vi "Navigation Loop.vi"(8 "error in (no error)":errorcluster) -> (0 "error out":errorcluster)   [LabVIEW 2016]
uses:
  Typedef/Filter Data.ctl
  <vilib>/Platform/TimedLoop/XDataNode/timing_clust.ctl
  <vilib>/Platform/TimedLoop/XDataNode/nitl_modes.ctl
  <vilib>/Platform/TimedLoop/XDataNode/wakeup.ctl
  <vilib>/Analysis/coordinate.llb/Wrap Angle (scalar).vi
  <vilib>/Analysis/baseanly.llb/Real Dot Product.vi
  <vilib>/Utility/file.llb/Read Delimited Spreadsheet (DBL).vi
  <vilib>/Utility/error.llb/Error Cluster From Error Code.vi
  Shared resoruces/Front Panel Control Variables.vi
  Shared resoruces/Navigation Variables.vi
  <vilib>/addons/control/pid/pid.llb/PID (DBL).vi
  <vilib>/ErrorRing/Error Ring.xnode
  <vilib>/platform/TimedLoop/XDataNode/XDataNode.xnode
  <vilib>/Platform/TimedLoop/XDataNode/XDNodeRunTimeDep.lvlib
  Shared resoruces/Shared resources RT.lvlib
  <vilib>/addons/control/pid/NI_PID_pid.lvlib
  <vilib>/Analysis/NI_AALBase.lvlib
  <vilib>/Analysis/NI_AAL_Angle.lvlib
  <vilib>/ptbypt/NI_PtbyPt.lvlib
panel:
  in  "Reference position":cluster{"Lat":dbl, "Long":dbl}={"Lat"=57.731096, "Long"=12.086851}
  in  "Heading PID gains":T1={"proportional gain (Kc)"=0.2, "integral time (Ti, min)"=0.0, "derivative time (Td, min)"=0.0} {"derivative time (Td, min)" format="%.3f"; "integral time (Ti, min)" format="%.3f"; "proportional gain (Kc)" format="%.3f"}
  in  "Lateral PID Gains":T1={"proportional gain (Kc)"=5.0, "integral time (Ti, min)"=600.0, "derivative time (Td, min)"=0.0} {"derivative time (Td, min)" format="%.3f"; "integral time (Ti, min)" format="%.3f"; "proportional gain (Kc)" format="%.3f"}
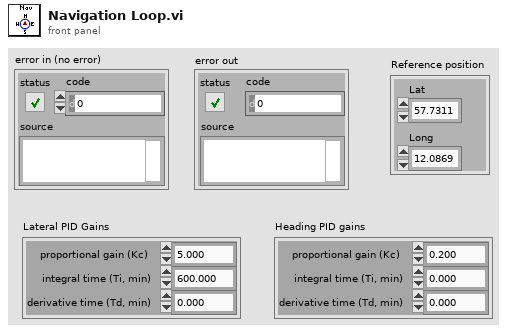
[diagram p1: front panel]
types:
  T1 = cluster{"proportional gain (Kc)":dbl, "integral time (Ti, min)":dbl, "derivative time (Td, min)":dbl}
  T2 = typedef "Filter Data.ctl" = cluster{"Yaw":dbl, "Lat":dbl, "Long":dbl}
  T3 = typedef "XDNodeRunTimeDep.lvlib/timing_clust.ctl" = cluster{"Expected End [f-1]":u64, "Actual End [f-1]":u64, "Finished Late? [f-1]":bool, "Expected End [i-1]":u64, "Actual End [i-1]":u64, "Finished Late? [i-1]":bool, "Expected Start [i]":u64, "Actual Start [i]":u64, "Expected Start [f]":u64, "Actual Start [f]":u64, "Source Name":string, "Structure Name":string, "Period":i64, "Deadline":i64, "Offset":i64, "Start":i64, "Priority":i32, "Timeout":i32, "Mode":T4, "Wakeup Reason":T5, "Error":errorcluster, "Source Type":string, "Secondary Source Type":string, "Global End Time":u64, "Global Start Time":u64, "Frame Duration":u64, "Iteration Duration":u64, "Assigned CPU":i32, "I/O Scan Engine Mode":u32}
  T4 = typedef "XDNodeRunTimeDep.lvlib/nitl_modes.ctl" = enum32{"No Change", "Process missed periods, maintain original phase", "Discard missed periods, maintain original phase", "Process missed periods, ignore original phase", "Discard missed periods, ignore original phase"}
  T5 = typedef "XDNodeRunTimeDep.lvlib/wakeup.ctl" = enum32{"Normal", "Aborted", "Asynchronous wakeup", "Timing source error", "Timed loop error", "Timeout"}
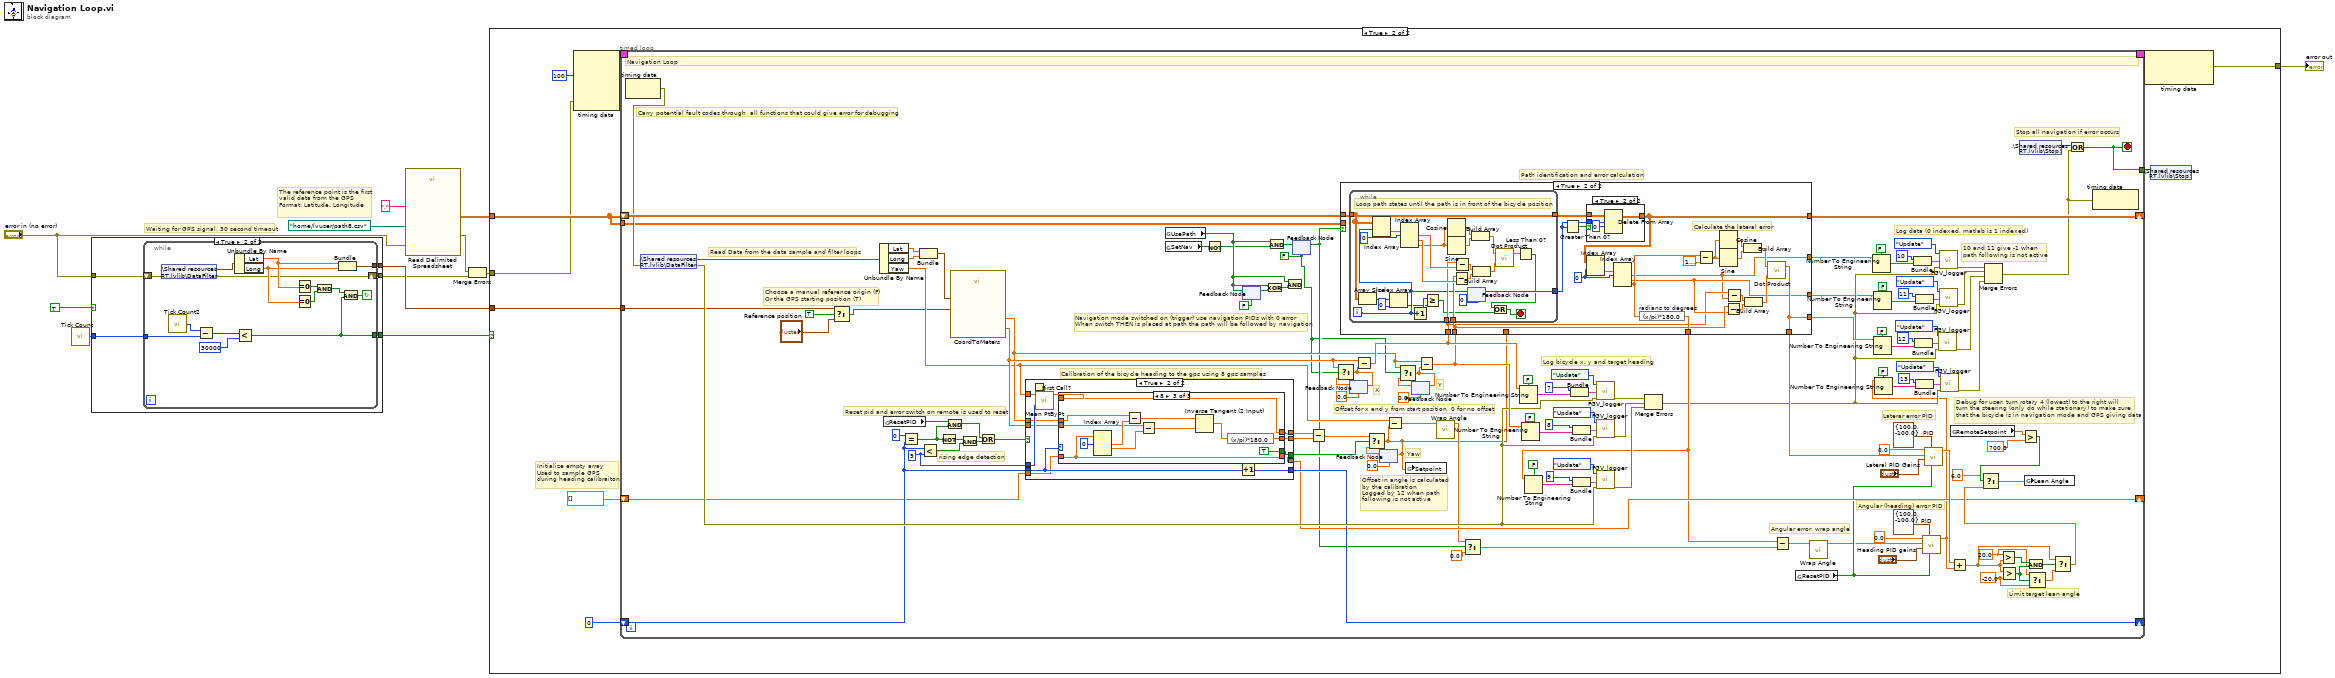
[diagram p0: block diagram]
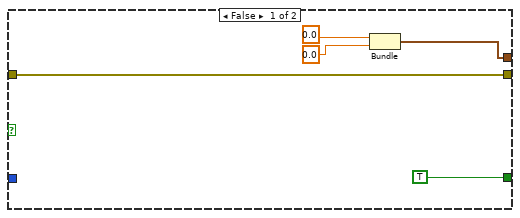
[diagram p2: hidden frame]
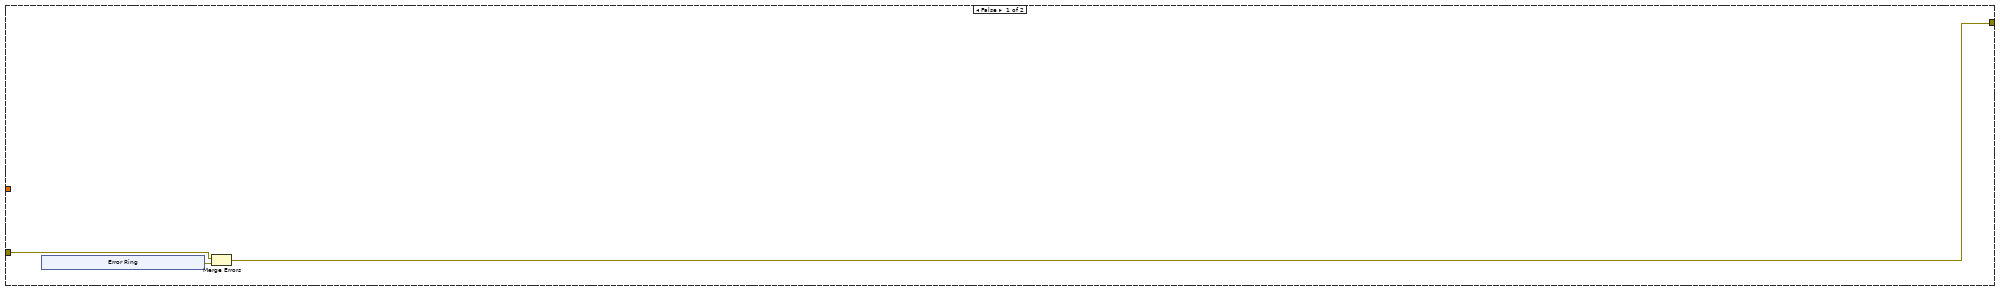
[diagram p3: hidden frame]
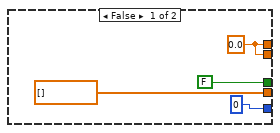
[diagram p4: hidden frame]
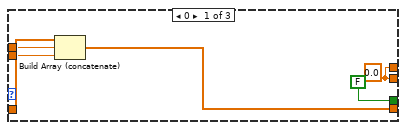
[diagram p5: hidden frame]
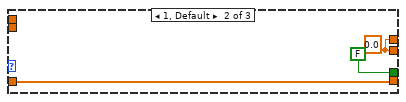
[diagram p6: hidden frame]
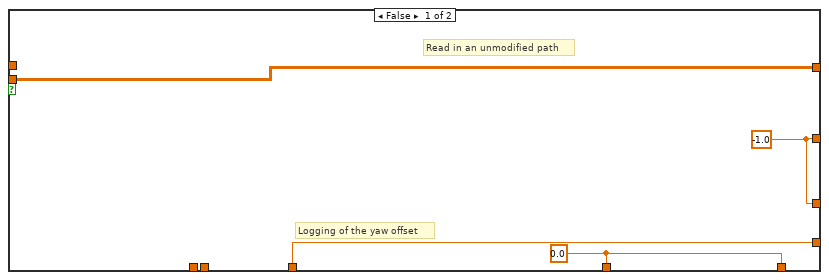
[diagram p7: hidden frame]
diagram:
  # "Waiting for GPS signal, 30 second timeout"
  # "The reference point is the first valid data from the GPS\nFormat: Latitude, Longitude"
  n1 = call "Tick Count"() -> ("Tick Count(mSec)"=w3:u32)
  n2 = case shown="True" TRUE {
    tunnel: "error in (no error)" -> [w17 w22]
    tunnel: [w16 w21] -> w10
    tunnel: [w17 w20] -> w7
    tunnel: w3 -> [_ w19]
    tunnel: [TRUE w18] -> w1
    frame False {
      n3 = Bundle(0.0, 0.0) -> (w16:cluster{dbl, dbl})  [unwired: 1 in]
    }
    frame True {
      n4 = while {
        shift-right: [w31] -> w20
        shift-left: w22 -> [w30]
        tunnel: [w34] -> w21
        tunnel: w19 -> [w26]
        tunnel: [w23] -> w18
        stop <- w28 continue-if-true
        n5 = shared-variable ".\\Shared resources RT.lvlib\\DataFilter"(error in=w30) -> (w35:T2, error out=w31:errorcluster)
        n6 = call "Tick Count2"() -> ("Tick Count(mSec)"=w27:u32)
        n7 = Subtract(x=w27, y=w26) -> (x-y=w25:u32)
        n8 = Unbundle By Name(w35) -> ("Lat"=w33:dbl, "Long"=w32:dbl)
        n9 = Less?(x=w25, y=u32 30000) -> (x < y?=w23:bool)
        n10 = Equal To 0?(x=w33) -> (x = 0?=w37:bool)
        n11 = Equal To 0?(x=w32) -> (x = 0?=w36:bool)
        n12 = And(x=w37, y=w36) -> (x .and. y?=w29:bool)
        n13 = Bundle("Lat"=w33, "Long"=w32) -> (w34:cluster{"Lat":dbl, "Long":dbl})  [unwired: 1 in]
        n14 = And(x=w29, y=w23) -> (x .and. y?=w28:bool)
      }
    }
  }
  n15 = call-poly <vilib>:"Read Delimited Spreadsheet.vi"("file path (dialog if empty)"=path "/home/lvuser/path8.csv", "error in (no error)"="error in (no error)", "delimiter (\\t)"="," ("delimiter (\\t)")) -> ("all rows"=w6:dbl[][], "error out"=w8:errorcluster)  [unwired: 7 in, 4 out]
  n16 = Merge Errors(w8, w7) -> (w9:errorcluster)
  n17 = case shown="True" w1 {
    tunnel: [w38 w49] -> w11
    tunnel: w10 -> [_ w53]
    tunnel: w9 -> [w40 w50]
    tunnel: w6 -> [_ w51]
    frame False {
      n18 = xnode "Error Ring"() -> ("error out"=w39:errorcluster)
      n19 = Merge Errors(w40, w39) -> (w38:errorcluster)
    }
    frame True {
      # "Initialize empty array\nUsed to sample GPS \nduring heading calibraiton"
      n20 = node-c288(i64 100 ("Period"), w50) -> (w55:T3)  [unwired: 3 in]
      n21 = timed-loop {
        shift-right: [w187] -> _
        shift-left: w51 -> [w186]
        tunnel: [w184] -> w52
        tunnel: w53 -> [w62]
        timing: w55 -> [_]
        timing-out: [_] -> w54
        tunnel: w51 -> [w108]
        shift-right: [w96] -> _
        shift-left: 0 -> [w87]
        shift-right: [w84] -> _
        shift-left: dbl[] [] -> [w83]
        stop <- w184 stop-if-true
        w86 = 9
        w102 = -20.0
        w103 = 20.0
        w57 = FALSE
        # "10 and 11 give -1 when\npath following is not active"
        # "Log bicycle x, y and target heading"
        # "Stop all navigation if error occurs"
        # "Carry potential fault codes through  all functions that could give error for debugging"
        # "Read Data from the data sample and filter loops"
        # "Laterar error PID"
        # "Angular (heading) error PID"
        # "Debug for user, turn rotary 4 (lowest) to the right will \nturn the steering (only do while stationary) to make sure \nthat the bicycle is in navigation mode and GPS giving data"
        # "Navigation mode switched on (trigger) use navigation PIDs with 0 error\nWhen switch THEN is placed at path the path will be followed by navigation"
        # "Offset in angle is calculated\nby the calibration\nLogged by 12 when path \nfollowing is not active"
        # "rising edge detection"
        # "Reset pid and error switch on remote is used to reset"
        # "Calibration of the bicycle heading to the gps using 8 gps samples"
        # "Log data (0 indexed, matlab is 1 indexed)"
        # "Angular error, wrap angle"
        # "Limit target lean angle"
        # "Path identification and error calculation"
        # "Choose a manual reference origin (F)\nOr the GPS starting position (T)"
        # "Yaw"
        # "Y"
        # "X"
        # "Offset for x and y from start position, 0 for no offset"
        # "Navigation Loop"
        n22 = node-c288() -> (w183:errorcluster)  [unwired: 1 in]
        n23 = shared-variable ".\\Shared resources RT.lvlib\\DataFilter"(error in=w183) -> (w185:T2, error out=w116:errorcluster)
        n24 = Select(t=w62, s=TRUE, f="Reference position") -> (s? t:f=w61:cluster{"Lat":dbl, "Long":dbl})
        n25 = Unbundle By Name(w185) -> ("Lat"=w115:dbl, "Long"=w114:dbl, "Yaw"=w72:dbl)
        n26 = global read "Front Panel Control Variables.vi" "ResetPID"() -> (w79:bool)
        n27 = Equal?(x=0, y=w87) -> (x = y?=w89:bool)
        n28 = Bundle("Lat"=w115, "Long"=w114) -> (w113:cluster{"Lat":dbl, "Long":dbl})  [unwired: 1 in]
        n29 = Less?(x=w87, y=w86) -> (x < y?=w90:bool)
        n30 = Not(x=w89) -> (.not. x?=w88:bool)
        n31 = And(x=w79, y=w89) -> (x .and. y?=w81:bool)
        n32 = call "CoordToMeters.vi"("Ref Point"=w61, "GPS position"=w113) -> ("X"=w95:dbl, "Y"=w94:dbl)  [unwired: 8 in]
        n33 = And(x=w88, y=w90) -> (x .and. y?=w92:bool)
        n34 = Or(x=w81, y=w92) -> (x .or. y?=w91:bool)
        n35 = case shown="True" w91 {
          tunnel: [FALSE w204] -> w98
          tunnel: [w190 w203] -> w97
          tunnel: w87 -> [_ w196]
          tunnel: [0 w197] -> w96
          tunnel: w95 -> [_ w192]
          tunnel: w94 -> [_ w193]
          tunnel: w86 -> [_ w200]
          tunnel: [w190 w202] -> w85
          tunnel: w72 -> [_ w199]
          tunnel: w83 -> [_ w195]
          tunnel: [dbl[] [] w194] -> w84
          frame False {
            w190 = 0.0
          }
          frame True {
            n36 = First Call?() -> (First Call?: T/F=w201:bool)
            n37 = call <vilib>:"Mean PtByPt.vi"("x"=w199, "sample length"=w200, "initialize"=w201) -> ("mean"=w198:dbl)  [unwired: 1 in, 1 out]
            n38 = case shown="8" w196 {
              tunnel: [FALSE FALSE TRUE] -> w204
              tunnel: [w209 w212 w223] -> w203
              tunnel: [w209 w212 w222] -> w202
              tunnel: w198 -> [_ _ w222]
              tunnel: w195 -> [w208 w211 w218]
              tunnel: [w205 w211 w218] -> w194
              tunnel: w193 -> [w207 _ w217]
              tunnel: w192 -> [w206 _ w215]
              frame 0 {
                w209 = 0.0
                n39 = Build Array (concatenate)(w208, w207, w206) -> (w205:dbl[])
              }
              frame 1, Default {
                w212 = 0.0
              }
              frame 8 {
                n40 = Index Array(array=w218, index #1=0) -> (element #1=w216:dbl, element #2=w214:dbl)  [unwired: 2 in, 1 out]
                n41 = Subtract(x=w217, y=w216) -> (x-y=w220:dbl)
                n42 = Subtract(x=w215, y=w214) -> (x-y=w219:dbl)
                n43 = Inverse Tangent (2 Input)(1:w219, 2:w220) -> (0:w225:dbl)
                n44 = expression code="(x/pi)*180.0" ("radians to degrees")(w225) -> (w223:dbl)
              }
            }
            n45 = Increment(x=w196) -> (x+1=w197:i32)
          }
        }
        n46 = global read "Navigation Variables.vi" "UsePath"() -> (w135:bool)
        n47 = global read "Navigation Variables.vi" "SetNav"() -> (w177:bool)
        n48 = Not(x=w177) -> (.not. x?=w119:bool)
        n49 = feedback #1(FALSE) -> (w136:bool)
        n50 = feedback-in #1(w135) -> ()
        n51 = Exclusive Or(1:w136, 2:w135) -> (0:w138:bool)
        n52 = And(x=w135, y=w119) -> (x .and. y?=w134:bool)
        n53 = And(x=w135, y=w138) -> ()  [unwired: 1 out]
        n54 = feedback #2(w57) -> (w58:bool)
        n55 = feedback-in #2(w134) -> ()
        n56 = Subtract(x=w85, y=w97) -> (x-y=w107:dbl)
        n57 = feedback #3(0.0 ("Roll")) -> (w170:dbl)
        n58 = Select(t=w95, s=w57, f=w170) -> (s? t:f=w168:dbl)
        n59 = feedback-in #3(w168) -> ()
        n60 = Subtract(x=w95, y=w168) -> (x-y=w123:dbl)
        n61 = feedback #4(0.0 ("Roll")) -> (w109:dbl)
        n62 = Select(t=w107, s=w98, f=w109) -> (s? t:f=w71:dbl)
        n63 = feedback-in #4(w71) -> ()
        n64 = Subtract(x=w72, y=w71) -> (x-y=w78:dbl)
        n65 = global write "Navigation Variables.vi" "Setpoint"(w71) -> ()
        n66 = feedback #5(0.0 ("Roll")) -> (w165:dbl)
        n67 = Select(t=w94, s=w57, f=w165) -> (s? t:f=w166:dbl)
        n68 = feedback-in #5(w166) -> ()
        n69 = Subtract(x=w94, y=w166) -> (x-y=w122:dbl)
        n70 = case shown="True" w58 {
          tunnel: w186 -> [_ w250]
          tunnel: [w229 w246] -> w187
          tunnel: [w227 w251] -> w76
          tunnel: w108 -> [w229 _]
          tunnel: w123 -> [_ w231]
          tunnel: w122 -> [_ w233]
          tunnel: [w227 w234] -> w145
          tunnel: [w228 w230] -> w154
          tunnel: [w228 w232] -> w56
          tunnel: w71 -> [w226 _]
          tunnel: [w226 w234] -> w82
          frame False {
            w228 = -1.0 ("index (row)")
            w227 = 0.0 ("index (row)")
            # "Logging of the yaw offset"
            # "Read in an unmodified path"
          }
          frame True {
            w245 = 0 ("index (row)")
            # "Calculate the lateral error"
            n71 = while {
              tunnel: w250 -> [w271]
              tunnel: w231 -> [w268]
              tunnel: w233 -> [w267]
              tunnel: [w271] -> w249
              tunnel: [w257] -> w235
              i -> [w258]
              stop <- w273 stop-if-true
              # "Loop path states until the path is in front of the bicycle position"
              n72 = Array Size(array=w271) -> (size(s)=w275:i32[])
              n73 = Index Array(array=w271, index (row)=w258) -> (element=w276:dbl[])  [unwired: 1 in]
              n74 = Index Array(array=w275, index=0 ("index (row)")) -> (element=w253:i32)
              n75 = Index Array(array=w276, index #1=0 ("index (row)")) -> (element #1=w270:dbl, element #2=w269:dbl, element #3=w262:dbl)  [unwired: 2 in]
              n76 = Increment(x=w258) -> (x+1=w254:i32)
              n77 = Greater Or Equal?(x=w254, y=w253) -> (x >= y?=w252:bool)
              n78 = Cosine(x=w262) -> (cos(x)=w263:dbl)
              n79 = Sine(x=w262) -> (sin(x)=w264:dbl)
              n80 = Subtract(x=w267, y=w269) -> (x-y=w265:dbl)
              n81 = Subtract(x=w268, y=w270) -> (x-y=w266:dbl)
              n82 = feedback-in #6(w258) -> ()
              n83 = feedback #6(0 ("index (row)")) -> (w257:i32)
              n84 = Build Array(w263, w264) -> (w261:dbl[])
              n85 = Build Array(w266, w265) -> (w260:dbl[])
              n86 = call-poly <vilib>:"Dot Product.vi"("Y Vector"=w260, "X Vector"=w261) -> ("X * Y"=w259:dbl)  [unwired: 1 out]
              n87 = Less Than 0?(x=w259) -> (x < 0?=w255:bool)
              n88 = Or(x=w255, y=w252) -> (x .or. y?=w273:bool)
            }
            n89 = Greater Than 0?(x=w235) -> (x > 0?=w248:bool)
            n90 = case shown="True" w248 {
              tunnel: [w277 w280] -> w246
              tunnel: w249 -> [w277 w279]
              tunnel: w235 -> [_ w278]
              frame False {
              }
              frame True {
                n91 = Delete From Array(array=w279, length=w278, index (row)=0) -> (array with subset deleted=w280:dbl[][])  [unwired: 1 in, 1 out]
              }
            }
            n92 = Index Array(array=w246, index (row)=w245) -> (element=w247:dbl[])  [unwired: 1 in]
            n93 = Index Array(array=w247, index #1=w245) -> (element #1=w230:dbl, element #2=w232:dbl, element #3=w238:dbl)  [unwired: 2 in]
            n94 = expression code="(x/pi)*180.0" "radians to degrees"(w238) -> (w251:dbl)
            n95 = Subtract(x=w238, y=1.5707963267948966) -> (x-y=w237:dbl)
            n96 = Cosine(x=w237) -> (cos(x)=w241:dbl)
            n97 = Sine(x=w237) -> (sin(x)=w242:dbl)
            n98 = Subtract(x=w233, y=w232) -> (x-y=w243:dbl)
            n99 = Subtract(x=w231, y=w230) -> (x-y=w244:dbl)
            n100 = Build Array(w241, w242) -> (w240:dbl[])
            n101 = Build Array(w244, w243) -> (w239:dbl[])
            n102 = call-poly <vilib>:"Dot Product.vi"("Y Vector"=w239, "X Vector"=w240) -> ("X * Y"=w234:dbl)  [unwired: 1 out]
          }
        }
        n103 = call-poly <vilib>:"Wrap Angle.vi"("angle in"=w78) -> ("angle out"=w77:dbl)  [unwired: 9 in, 1 out]
        n104 = Select(t=w77, s=w58, f=0.0 ("Roll")) -> (s? t:f=w112:dbl)
        n105 = Number To Engineering String(1:FALSE ("use system decimal point (T)"), 4:w123) -> (0:w133:string)  [unwired: 2 in]
        n106 = Number To Engineering String(1:FALSE ("use system decimal point (T)"), 4:w122) -> (0:w124:string)  [unwired: 2 in]
        n107 = Number To Engineering String(1:FALSE ("use system decimal point (T)"), 4:w76) -> (0:w174:string)  [unwired: 2 in]
        n108 = Bundle(7, w133) -> (w132:cluster{i32, string})  [unwired: 1 in]
        n109 = Bundle(8, w124) -> (w125:cluster{i32, string})  [unwired: 1 in]
        n110 = Bundle(9, w174) -> (w175:cluster{i32, string})  [unwired: 1 in]
        n111 = call "FGV_logger.vi"("error in"=w116, 9:w132, "Command"=enum16{"Update", "Log", "Init"}."Update") -> ("error out"=w120:errorcluster)  [unwired: 8 in]
        n112 = call "FGV_logger.vi"("error in"=w116, 9:w125, "Command"=enum16{"Update", "Log", "Init"}."Update") -> ("error out"=w121:errorcluster)  [unwired: 8 in]
        n113 = call "FGV_logger.vi"("error in"=w116, 9:w175, "Command"=enum16{"Update", "Log", "Init"}."Update") -> ("error out"=w171:errorcluster)  [unwired: 8 in]
        n114 = Merge Errors(w120, w121, w171) -> (w64:errorcluster)
        n115 = Subtract(x=w76, y=w112) -> (x-y=w75:dbl)
        n116 = global read "Front Panel Control Variables.vi" "ResetPID"() -> (w80:bool)
        n117 = call-poly <vilib>:"Wrap Angle.vi"("angle in"=w75) -> ("angle out"=w74:dbl)  [unwired: 9 in, 1 out]
        n118 = Number To Engineering String(1:FALSE ("use system decimal point (T)"), 4:w154) -> (0:w155:string)  [unwired: 2 in]
        n119 = Number To Engineering String(1:FALSE ("use system decimal point (T)"), 4:w82) -> (0:w151:string)  [unwired: 2 in]
        n120 = Number To Engineering String(1:FALSE ("use system decimal point (T)"), 4:w56) -> (0:w164:string)  [unwired: 2 in]
        n121 = Bundle(10, w155) -> (w156:cluster{i32, string})  [unwired: 1 in]
        n122 = Bundle(12, w151) -> (w150:cluster{i32, string})  [unwired: 1 in]
        n123 = Bundle(11, w164) -> (w163:cluster{i32, string})  [unwired: 1 in]
        n124 = call-poly <vilib>:"PID.vi"("reinitialize? (F)"=w80, "output range"=cluster{"output high":dbl, "output low":dbl} {"output high"=100.0, "output low"=-100.0}, "PID gains"="Heading PID gains", "process variable"=w74, "setpoint"=0.0 ("Roll")) -> ("output"=w63:dbl)  [unwired: 5 in, 1 out]
        n125 = Number To Engineering String(1:FALSE ("use system decimal point (T)"), 4:w63) -> (0:w70:string)  [unwired: 2 in]
        n126 = Bundle(13, w70) -> (w69:cluster{i32, string})  [unwired: 1 in]
        n127 = call-poly <vilib>:"PID.vi"("reinitialize? (F)"=w80, "output range"=cluster{"output high":dbl, "output low":dbl} {"output high"=100.0, "output low"=-100.0}, "PID gains"="Lateral PID Gains", "process variable"=w145, "setpoint"=0.0 ("Roll")) -> ("output"=w178:dbl)  [unwired: 5 in, 1 out]
        n128 = call "FGV_logger.vi"("error in"=w64, 9:w150, "Command"=enum16{"Update", "Log", "Init"}."Update") -> ("error out"=w146:errorcluster)  [unwired: 8 in]
        n129 = call "FGV_logger.vi"("error in"=w64, 9:w156, "Command"=enum16{"Update", "Log", "Init"}."Update") -> ("error out"=w153:errorcluster)  [unwired: 8 in]
        n130 = call "FGV_logger.vi"("error in"=w64, 9:w163, "Command"=enum16{"Update", "Log", "Init"}."Update") -> ("error out"=w152:errorcluster)  [unwired: 8 in]
        n131 = call "FGV_logger.vi"("error in"=w64, 9:w69, "Command"=enum16{"Update", "Log", "Init"}."Update") -> ("error out"=w65:errorcluster)  [unwired: 8 in]
        n132 = global read "Navigation Variables.vi" "RemoteSetpoint"() -> (w143:dbl)
        n133 = Add(x=w178, y=w63) -> (x+y=w100:dbl)
        n134 = Merge Errors(w153, w152, w146, w65) -> (w117:errorcluster)
        n135 = Greater?(x=w103, y=w100) -> (0:w106:bool)
        n136 = Greater?(x=w100, y=w102) -> (0:w104:bool)
        n137 = shared-variable ".\\Shared resources RT.lvlib\\Stop!"() -> (w118:bool)  [unwired: 1 in, 1 out]
        n138 = Greater?(x=w143, y=700.0 ("Roll")) -> (0:w140:bool)
        n139 = And(x=w106, y=w104) -> (x .and. y?=w105:bool)
        n140 = Select(t=w103, s=w104, f=w102) -> (s? t:f=w101:dbl)
        n141 = Select(t=w100, s=w105, f=w101) -> (s? t:f=w99:dbl)
        n142 = Select(t=6.0 ("Roll"), s=w140, f=w99) -> (s? t:f=w141:dbl)
        n143 = global write "Navigation Variables.vi" "Lean Angle"(w141) -> ()
        n144 = Or(x=w118, y=w117) -> (x .or. y?=w184:bool)
        n145 = node-c288(w117) -> ()  [unwired: 1 out]
      }
      n146 = node-c288(w54) -> (w49:errorcluster)  [unwired: 1 out]
      n147 = shared-variable ".\\Shared resources RT.lvlib\\Stop!"(w52) -> ()  [unwired: 1 in, 1 out]
    }
  }
  "error out" <- w11
